vi "DisplaySpeedDisplay_171213.vi"(11 "Display Speed":dbl) -> (3 "PlayBackSpeedDisplay":string)   [LabVIEW 2016]
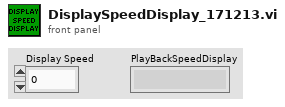
[diagram p1: front panel]
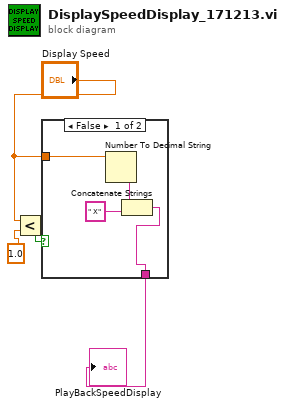
[diagram p0: block diagram]
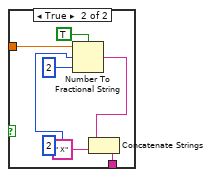
[diagram p2: hidden frame]
diagram:
  n1 = Less?(x="Display Speed", y=1.0) -> (x < y?=w1:bool)
  n2 = case shown="False" w1 {
    tunnel: [w6 w10] -> w3
    tunnel: "Display Speed" -> [w5 w9]
    frame False {
      n3 = Number To Decimal String(number=w5) -> (decimal integer string=w8:string)  [unwired: 1 in]
      n4 = Concatenate Strings(w8, " X" ("string")) -> (w6:string)
    }
    frame True {
      n5 = Number To Fractional String(use system decimal point (T)=TRUE, number=w9, width (-)=i16 2, precision (6)=i16 2) -> (F-format string=w11:string)
      n6 = Concatenate Strings(w11, " X" ("string")) -> (w10:string)
    }
  }
  "PlayBackSpeedDisplay" <- w3
